vi "Append To Log.vi"(8 "error in (no error)":cluster{"状态":bool, "代码":i32, "源":string} caption="错误输入（无错误）", 10 "字符串":string, 11 "冷却器备用UI输入":refnum<class "Programmatic Controller.lvclass">) -> (0 "error out":cluster{"状态":bool, "代码":i32, "源":string} caption="错误输出")   [LabVIEW 2015, in "Programmatic Controller.lvclass"]
doc: "给定一个消息，追加至当前记录文件。调用方负责按需要向文本添加行结束字符。"
uses:
  Programmatic Controller.lvclass
  Programmatic Controller.lvclass/Programmatic Controller.ctl
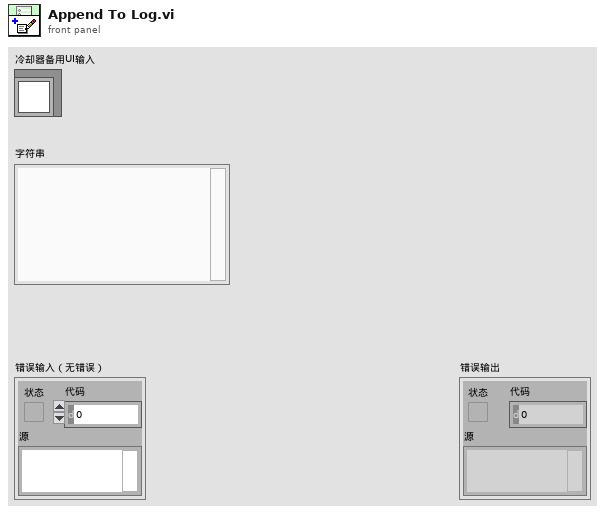
[diagram p1: front panel]
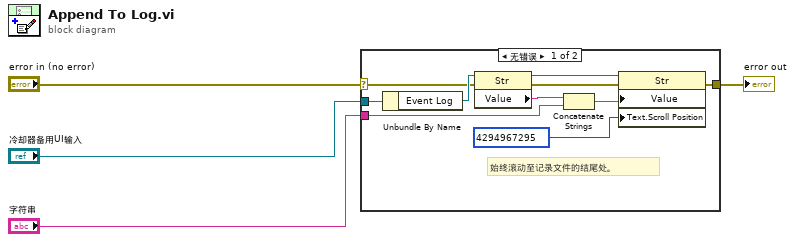
[diagram p0: block diagram]
diagram:
  n1 = case shown="无错误" "error in (no error)" {
    selector: "error in (no error)" -> [w10 w15]
    tunnel: [w9 w15] -> w3
    tunnel: "冷却器备用UI输入" -> [w14 _]
    tunnel: "字符串" -> [w7 _]
    frame No Error {
      # "始终滚动至记录文件的结尾处。"
      n2 = Unbundle By Name(w14) -> ("Event Log"=w13:refnum<vi>)
      n3 = property class="Str"(reference=w13, error in=w10) -> (reference out=w11:refnum<vi>, error out=w12:errorcluster, "Value"=w8:string)
      n4 = Concatenate Strings(w8, w7) -> (w6:string)
      n5 = property class="Str"(reference=w11, error in=w12, "Value"=w6, "Text.Scroll Position"=u32 4294967295) -> (error out=w9:errorcluster)  [unwired: 1 out]
    }
    frame Error {
    }
  }
  "error out" <- w3
